vi "Build Waveform Executables.vi"(6 "error in (no error)":errorcluster, 8 "Function":T1, 9 "Instrument Name":string) -> (0 "error out":errorcluster, 2 "Ids":string[](array[string]), 3 "Command Directors":refnum<class "CommandDirector.lvclass">[](array[class]))   [LabVIEW 2023]
uses:
  ResourceEnumerator/ResourceEnumerator.lvclass
  Measure/Measure Function.ctl
  HAF.lvlib
  CommandDirector/CommandDirector.lvclass
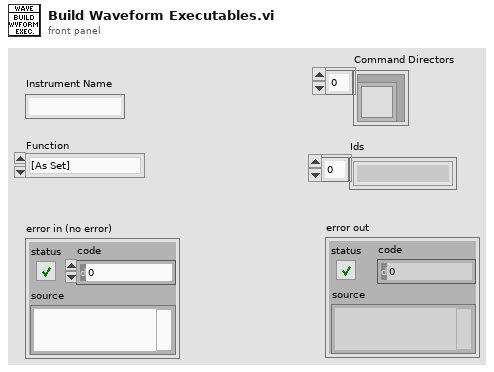
[diagram p1: front panel]
types:
  T1 = typedef "HAF.lvlib/Measure Function.ctl" = enum16{"[As Set]", "DC Voltage", "AC Voltage", "DC Current", "AC Current", "2-wire Resistance", "4-wire Resistance", "Diode", "Capacitance", "Temperature", "Continuity", "Frequency", "Period", "DC Voltage Ratio"}
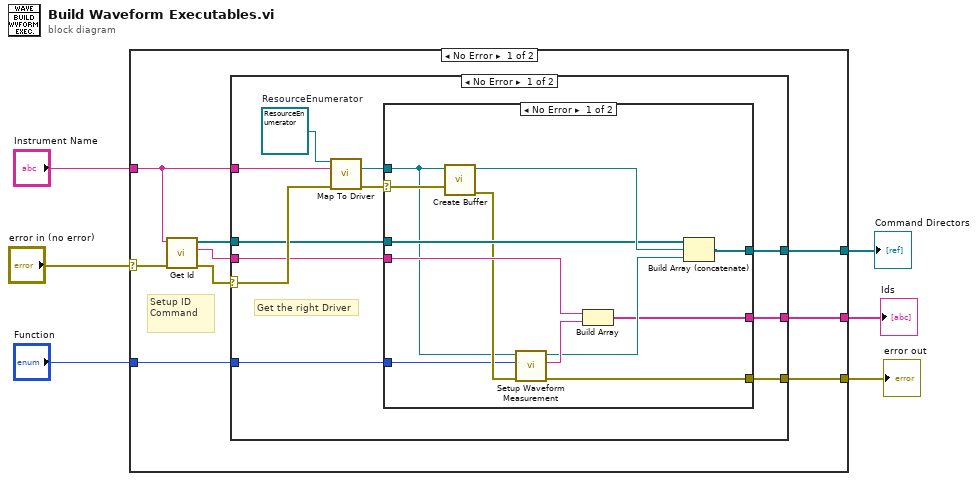
[diagram p0: block diagram]
diagram:
  n1 = case shown="No Error" "error in (no error)" {
    selector: "error in (no error)" -> [w15 w41]
    tunnel: "Instrument Name" -> [w11 _]
    tunnel: "Function" -> [w10 _]
    tunnel: [w9 _] -> w3
    tunnel: [w8 _] -> w2
    tunnel: [w7 w41] -> w1
    frame No Error {
      # "Setup ID Command"
      n2 = call "Get Id.vi"("error in (no error)"=w15, "Instrument Name"=w11) -> ("error out"=w14:errorcluster, "ID of IDN Command"=w12:string, "CommandDirectors"=w13:refnum<class "CommandDirector.lvclass">[])  [unwired: 6 in]
      n3 = case shown="No Error" w14 {
        selector: w14 -> [w24 w40]
        tunnel: w13 -> [w21 _]
        tunnel: w12 -> [w20 _]
        tunnel: w11 -> [w25 _]
        tunnel: w10 -> [w19 _]
        tunnel: [w18 _] -> w9
        tunnel: [w17 _] -> w8
        tunnel: [w16 w40] -> w7
        frame No Error {
          w26 = refnum<class "ResourceEnumerator.lvclass"> refnum  # ResourceEnumerator
          # "Get the right Driver"
          n4 = call-dynamic "Map To Driver.vi"("AbstractResourceEnumerator in"=w26, "Driver Name"=w25, "error in (no error)"=w24) -> ("Driver"=w23:refnum<class "Driver.lvclass">, "error out"=w22:errorcluster)  [unwired: 10 in, 1 out]
          n5 = case shown="No Error" w22 {
            selector: w22 -> [w38 w39]
            tunnel: w23 -> [w33 _]
            tunnel: w21 -> [w36 _]
            tunnel: w20 -> [w35 _]
            tunnel: w19 -> [w32 _]
            tunnel: [w29 _] -> w18
            tunnel: [w28 _] -> w17
            tunnel: [w27 w39] -> w16
            frame No Error {
              n6 = call "Create Buffer.vi"("error in (no error)"=w38, "Driver"=w33) -> ("error out"=w34:errorcluster, "CommandDirector"=w37:refnum<class "CommandDirector.lvclass">)  [unwired: 6 in]
              n7 = call "Setup Waveform Measurement.vi"("error in (no error)"=w34, "Function"=w32, "Driver"=w33) -> ("error out"=w27:errorcluster, "Id"=w31:string, "CommandDirector"=w30:refnum<class "CommandDirector.lvclass">)  [unwired: 4 in]
              n8 = Build Array(w35, w31) -> (w28:string[])
              n9 = Build Array (concatenate)(w36, w37, w30) -> (w29:refnum<class "CommandDirector.lvclass">[])
            }
            frame Error {
            }
          }
        }
        frame Error {
        }
      }
    }
    frame Error {
    }
  }
  "error out" <- w1
  "Ids" <- w2
  "Command Directors" <- w3
